vi "Setup Motors.vi"   [LabVIEW 2014]
uses:
  <vilib>/Rock Robotics/SystemInterfaces/Typedef/FPGA_TypedefDigitalModule.ctl
  <vilib>/Rock Robotics/SystemInterfaces/DIO/FPGA_DIOPWMChannel.ctl
  <vilib>/Rock Robotics/WPI/Joystick/WPI_JoystickDeviceEnum.ctl
  <vilib>/Rock Robotics/SystemInterfaces/Typedef/FPGA_TypedefAnalogModule.ctl
  <vilib>/Rock Robotics/SystemInterfaces/AI/FPGA_AIChannel.ctl
  <vilib>/Rock Robotics/WPI/Solenoid/WPI_SolenoidChannel.ctl
  <vilib>/Rock Robotics/SystemInterfaces/AI/FPGA_AIGyroChannel.ctl
  <vilib>/Rock Robotics/SystemInterfaces/Typedef/FPGA_TypedefAnalogModuleForGyro.ctl
  <vilib>/Rock Robotics/SystemInterfaces/DIO/FPGA_DIOChannel.ctl
  <vilib>/Rock Robotics/WPI/SafetyOutput/WPI_SafetyOutputConfigMenu.ctl
  <vilib>/Rock Robotics/WPI/MotorControl/WPI_MotorControlOpen Talon.vi
  <vilib>/Rock Robotics/WPI/Solenoid/WPI_SolenoidOpenSingle.vi
  <vilib>/Rock Robotics/WPI/Switch/WPI_SwitchOpenLimit.vi
  <vilib>/Rock Robotics/WPI/Counter/WPI_CounterDigitalInputToDigitalSource.vi
  Global Variables.vi
types:
  T1 = typedef "WPI_SafetyOutputConfigMenu.ctl" = enum16{"Enable", "Disable"}
  T2 = typedef "WPI_SolenoidChannel.ctl" = enum8{"Solenoid 0", "Solenoid 1", "Solenoid 2", "Solenoid 3", "Solenoid 4", "Solenoid 5", "Solenoid 6", "Solenoid 7", "Invalid"}
  T3 = typedef "FPGA_DIOChannel.ctl" = enum8{"DIO 0", "DIO 1", "DIO 2", "DIO 3", "DIO 4", "DIO 5", "DIO 6", "DIO 7", "DIO 8", "DIO 9", "DIO MXP 0", "DIO MXP 1", "DIO MXP 2", "DIO MXP 3", "DIO MXP 4", "DIO MXP 5", "DIO MXP 6", "DIO MXP 7", "DIO MXP 8", "DIO MXP 9", "DIO MXP 10", "DIO MXP 11", "DIO MXP 12", "DIO MXP 13", "DIO MXP 14", "DIO MXP 15", "Invalid"}
  T4 = typedef "FPGA_TypedefDigitalModule.ctl" = enum16{"Controller 1"}
  T5 = typedef "FPGA_TypedefAnalogModuleForGyro.ctl" = enum16{"Controller 1"}
  T6 = typedef "FPGA_AIGyroChannel.ctl" = enum8{"AI 0", "AI 1", "Invalid"}
  T7 = typedef "FPGA_DIOPWMChannel.ctl" = enum8{"PWM 0", "PWM 1", "PWM 2", "PWM 3", "PWM 4", "PWM 5", "PWM 6", "PWM 7", "PWM 8", "PWM 9", "PWM MXP 0", "PWM MXP 1", "PWM MXP 2", "PWM MXP 3", "PWM MXP 4", "PWM MXP 5", "PWM MXP 6", "PWM MXP 7", "PWM MXP 8", "PWM MXP 9", "Invalid"}
  T8 = typedef "FPGA_AIChannel.ctl" = enum8{"AI 0", "AI 1", "AI 2", "AI 3", "AI MXP 0", "AI MXP 1", "AI MXP 2", "AI MXP 3", "Invalid"}
  T9 = typedef "FPGA_TypedefAnalogModule.ctl" = enum16{"Controller 1"}
  T10 = typedef "WPI_JoystickDeviceEnum.ctl" = enum16{"USB 0", "USB 1", "USB 2", "USB 3", "USB 4", "USB 5"}
  T11 = typedef "WPI_MotorControlDeviceRef.ctl" = cluster{"DeviceStatus":errorcluster, "Type":T12, "PWM":cluster{"Controller":T4, "PWM Channel":T7, "DeadBand":T13}, "CAN":cluster{"Device Number":u8, "Control Mode":T14, "Semaphore":T15, "Max Vout":dbl, "TalonSRX Control Mode":T16}, "Invert":bool, "TransformRef":T17, "InvTransformRef":T17}
  T12 = typedef "WPI_MotorControlType.ctl" = enum16{"PWM", "CAN", "CANTalonSRX"}
  T13 = typedef "WPI_PWMDeadband.ctl" = cluster{"Name":string, "maxPositivePwm":i32, "minPositivePwm":i32, "centerPwm":i32, "maxNegativePwm":i32, "minNegativePwm":i32, "angularRange":u16}
  T14 = typedef "WPI_CANJaguar_ControlMode.ctl" = enum8{"Percent VBus", "Current", "Speed", "Position", "Voltage"}
  T15 = typedef "Semaphore RefNum" = refnum<k1>
  T16 = typedef "WPI_CANTalonSRX_APIControlMode.ctl" = enum8{"Percent VBus", "Speed", "Position", "Slave", "Unchanged / Invalid"}
  T17 = typedef "WPI_PWMTransform_ConPane.ctl" = refnum<vi>
  T18 = typedef "WPI_GyroDevRef.ctl" = cluster{"DevStatus":errorcluster, "Analog Module":T9, "Analog Channel":T8, "Offset":dbl, "Gain (VoltsPerDegree/Second)":dbl}
  T19 = typedef "WPI_SolenoidDevRef.ctl" = cluster{"DevStatus":errorcluster, "Pneumatics Control Module":u8, "Forward Solenoid Channel":T2, "Reverse Solenoid Channel":T2}
  T20 = typedef "WPI_SwitchDevRef.ctl" = cluster{"DevStatus":errorcluster, "DIO Channel":T3, "Controller":T4, "CntIndex":T21, "Normally Closed":bool}
  T21 = typedef "FPGA_CounterCtrSystemIndex.ctl" = enum8{"Ctr 0", "Ctr 1", "Ctr 2", "Ctr 3", "Ctr 4", "Ctr 5", "Ctr 6", "Ctr 7", "Invalid"}
  T22 = typedef "WPI_DigitalInputDevRef.ctl" = cluster{"DevStatus":errorcluster, "DIO Channel":T3, "Controller":T4}
  T23 = typedef "FPGA_CounterEncoderSourceConvertionLVSourceType.ctl" = cluster{"DevStatus":errorcluster, "AnalogTriggerMode?":bool, "DigitalMode":cluster{"Controller":T4, "DIO Channel":T24}, "AnalogTriggerMode":cluster{"AnalogTriggerIndex":T25, "OutputType":T26}}
  T24 = typedef "FPGA_DIODigitalSourceChannel.ctl" = enum8{"DIO 0", "DIO 1", "DIO 2", "DIO 3", "DIO 4", "DIO 5", "DIO 6", "DIO 7", "DIO 8", "DIO 9", "DIO MXP 0", "DIO MXP 1", "DIO MXP 2", "DIO MXP 3", "DIO MXP 4", "DIO MXP 5", "DIO MXP 6", "DIO MXP 7", "DIO MXP 8", "DIO MXP 9", "DIO MXP 10", "DIO MXP 11", "DIO MXP 12", "DIO MXP 13", "DIO MXP 14", "DIO MXP 15", "Disabled"}
  T25 = typedef "FPGA_AnalogTriggerIndex.ctl" = enum8{"Trig 0", "Trig 1", "Trig 2", "Trig 3", "Trig 4", "Trig 5", "Trig 6", "Trig 7", "Invalid"}
  T26 = typedef "FPGA_AnalogTriggerOutType.ctl" = enum16{"InWindow", "TriggerState", "Rising", "Falling"}
  T27 = typedef "WPI_AnalogChannelDevRef.ctl" = cluster{"DevStatus":errorcluster, "Controller":T9, "Analog Channel":T8}
  T28 = typedef "WPI_EncoderDevRef.ctl" = cluster{"DevStatus":errorcluster, "EncoderIndex":T29, "CounterIndex":T21, "DistancePerCount":dbl, "Decoding Type":T30}
  T29 = typedef "FPGA_EncoderIdx.ctl" = enum8{"Enc 0", "Enc 1", "Enc 2", "Enc 3", "Enc 4", "Enc 5", "Enc 6", "Enc 7", "Invalid"}
  T30 = typedef "WPI_EncoderType.ctl" = enum16{"1x", "2x", "4x"}
  T31 = typedef "WPI_JoystickDevRef.ctl" = cluster{"Device":T10}
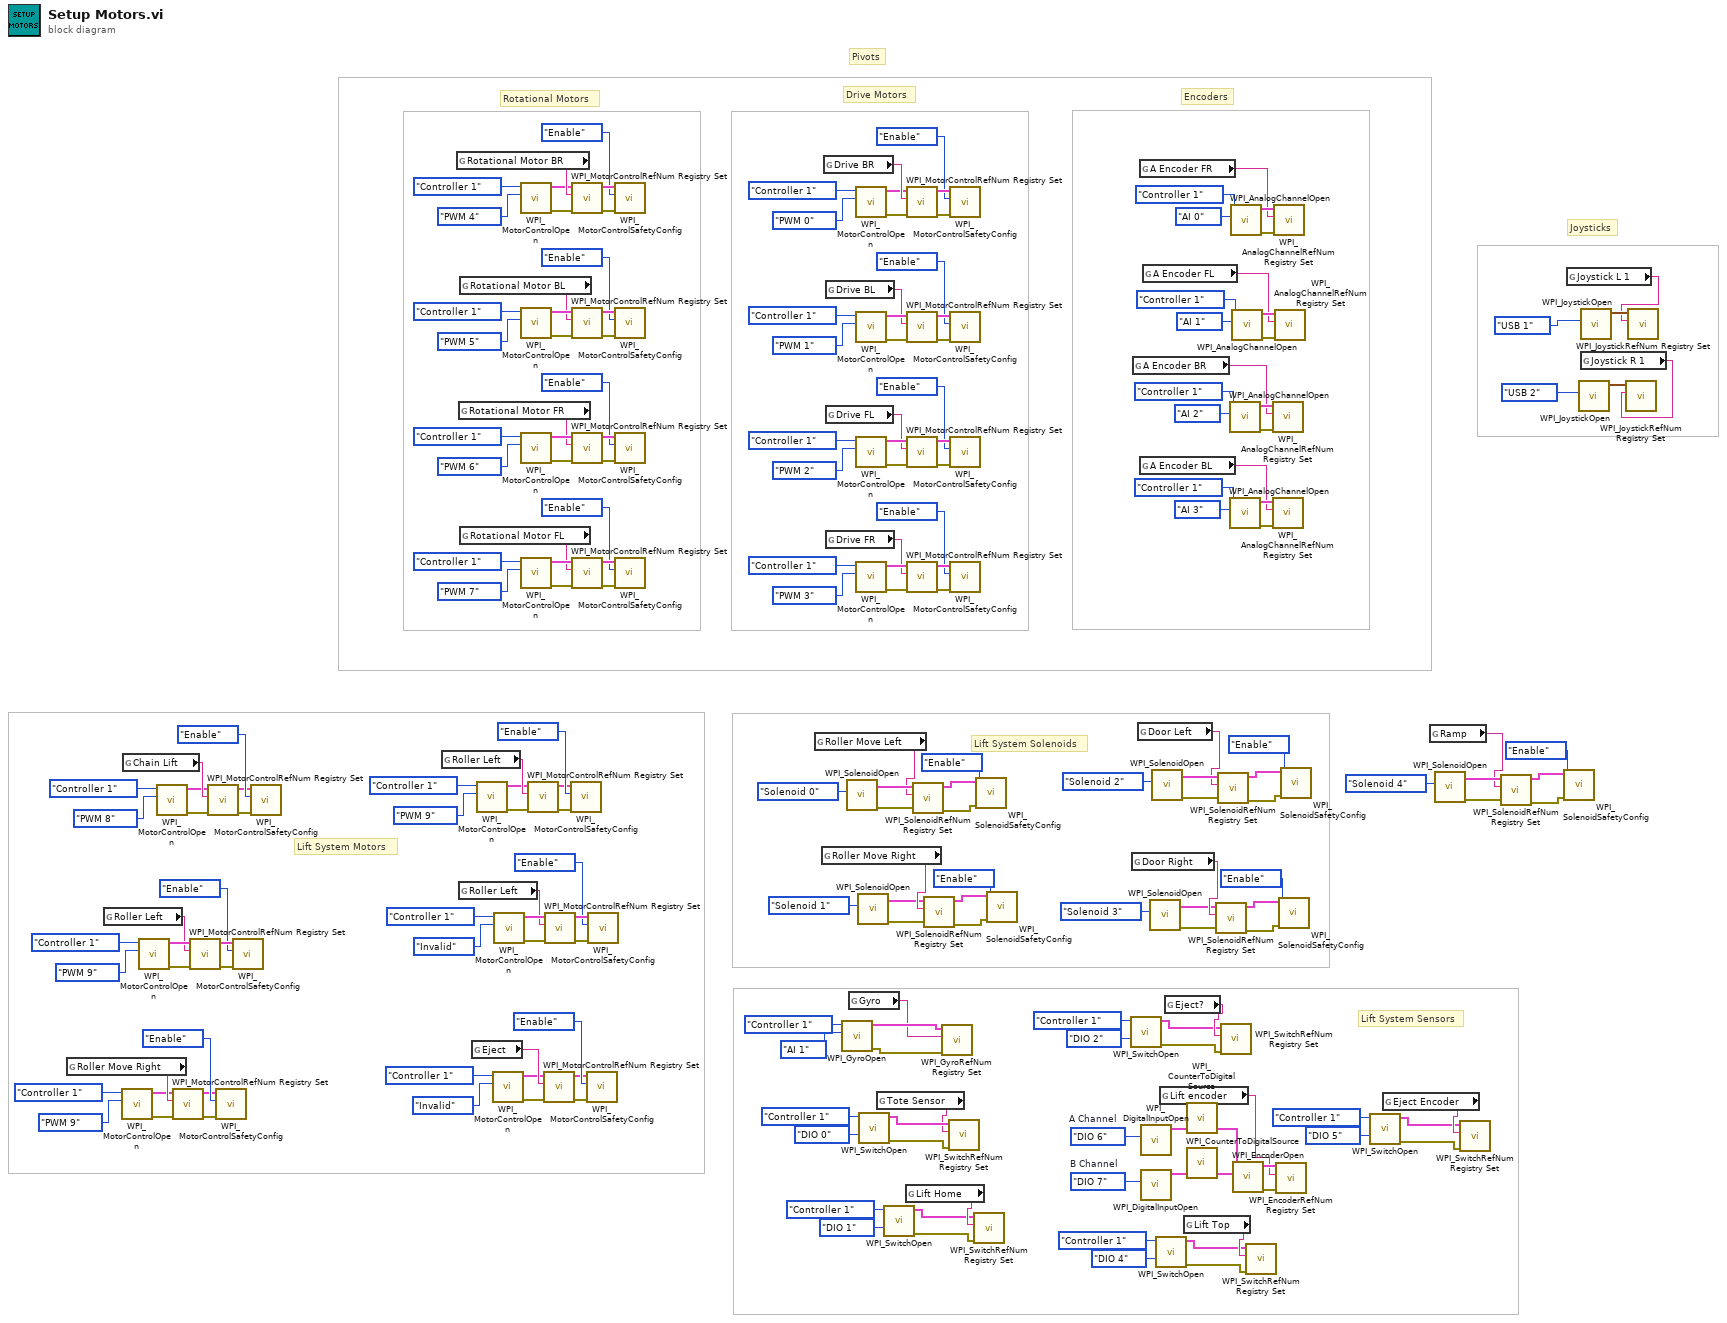
[diagram p0: block diagram]
diagram:
  w16 = FPGA_DIOChannel."DIO 7"  # B Channel
  w15 = FPGA_DIOChannel."DIO 6"  # A Channel
  # "Lift System Sensors"
  # "Lift System Solenoids"
  # "Lift System Motors"
  # "Encoders"
  # "Joysticks"
  # "Pivots"
  # "Rotational Motors"
  # "Drive Motors"
  n1 = global read "Global Variables.vi" "Roller Move Right"() -> (w105:string)
  n2 = global read "Global Variables.vi" "Roller Left"() -> (w108:string)
  n3 = call-poly <vilib>:"WPI_MotorControlOpen.vi"("PWM Channel"=FPGA_DIOPWMChannel."PWM 9", "Controller"=FPGA_TypedefDigitalModule."Controller 1") -> ("error out"=w100:errorcluster, "MotorControlDeviceRef"=w99:T11)  [unwired: 8 in]
  n4 = global read "Global Variables.vi" "Chain Lift"() -> (w121:string)
  n5 = call-poly <vilib>:"WPI_MotorControlOpen.vi"("PWM Channel"=FPGA_DIOPWMChannel."PWM 9", "Controller"=FPGA_TypedefDigitalModule."Controller 1") -> ("error out"=w113:errorcluster, "MotorControlDeviceRef"=w114:T11)  [unwired: 8 in]
  n6 = call-poly <vilib>:"WPI_MotorControlOpen.vi"("PWM Channel"=FPGA_DIOPWMChannel."PWM 8", "Controller"=FPGA_TypedefDigitalModule."Controller 1") -> ("error out"=w116:errorcluster, "MotorControlDeviceRef"=w115:T11)  [unwired: 8 in]
  n7 = call <vilib>:"WPI_MotorControlRefNum Registry Set.vi"("error in (no error)"=w100, "refnum name"=w105, "MotorControlDevRef"=w99) -> ("error out"=w102:errorcluster, "MotorControlDevRef"=w101:T11)  [unwired: 7 in]
  n8 = call <vilib>:"WPI_MotorControlRefNum Registry Set.vi"("error in (no error)"=w113, "refnum name"=w108, "MotorControlDevRef"=w114) -> ("error out"=w111:errorcluster, "MotorControlDevRef"=w112:T11)  [unwired: 7 in]
  n9 = call <vilib>:"WPI_MotorControlRefNum Registry Set.vi"("error in (no error)"=w116, "refnum name"=w121, "MotorControlDevRef"=w115) -> ("error out"=w118:errorcluster, "MotorControlDevRef"=w117:T11)  [unwired: 7 in]
  n10 = call <vilib>:"WPI_MotorControlSafetyConfig.vi"("error in (no error)"=w102, "mode"=WPI_SafetyOutputConfigMenu."Enable", "MotorControlDevRef"=w101) -> ()  [unwired: 7 in, 2 out]
  n11 = call <vilib>:"WPI_MotorControlSafetyConfig.vi"("error in (no error)"=w111, "mode"=WPI_SafetyOutputConfigMenu."Enable", "MotorControlDevRef"=w112) -> ()  [unwired: 7 in, 2 out]
  n12 = call <vilib>:"WPI_MotorControlSafetyConfig.vi"("error in (no error)"=w118, "mode"=WPI_SafetyOutputConfigMenu."Enable", "MotorControlDevRef"=w117) -> ()  [unwired: 7 in, 2 out]
  n13 = global read "Global Variables.vi" "Roller Left"() -> (w97:string)
  n14 = global read "Global Variables.vi" "Rotational Motor BR"() -> (w175:string)
  n15 = global read "Global Variables.vi" "Rotational Motor FR"() -> (w149:string)
  n16 = global read "Global Variables.vi" "Roller Left"() -> (w84:string)
  n17 = global read "Global Variables.vi" "Rotational Motor BL"() -> (w150:string)
  n18 = global read "Global Variables.vi" "Rotational Motor FL"() -> (w148:string)
  n19 = global read "Global Variables.vi" "Eject"() -> (w81:string)
  n20 = call-poly <vilib>:"WPI_MotorControlOpen.vi"("PWM Channel"=FPGA_DIOPWMChannel."PWM 9", "Controller"=FPGA_TypedefDigitalModule."Controller 1") -> ("error out"=w92:errorcluster, "MotorControlDeviceRef"=w91:T11)  [unwired: 8 in]
  n21 = call-poly <vilib>:"WPI_MotorControlOpen.vi"("PWM Channel"=FPGA_DIOPWMChannel."Invalid", "Controller"=FPGA_TypedefDigitalModule."Controller 1") -> ("error out"=w76:errorcluster, "MotorControlDeviceRef"=w75:T11)  [unwired: 8 in]
  n22 = call-poly <vilib>:"WPI_MotorControlOpen.vi"("PWM Channel"=FPGA_DIOPWMChannel."Invalid", "Controller"=FPGA_TypedefDigitalModule."Controller 1") -> ("error out"=w89:errorcluster, "MotorControlDeviceRef"=w90:T11)  [unwired: 8 in]
  n23 = call-poly <vilib>:"WPI_MotorControlOpen.vi"("PWM Channel"=FPGA_DIOPWMChannel."PWM 4", "Controller"=FPGA_TypedefDigitalModule."Controller 1") -> ("error out"=w173:errorcluster, "MotorControlDeviceRef"=w174:T11)  [unwired: 8 in]
  n24 = call-poly <vilib>:"WPI_MotorControlOpen.vi"("PWM Channel"=FPGA_DIOPWMChannel."PWM 5", "Controller"=FPGA_TypedefDigitalModule."Controller 1") -> ("error out"=w167:errorcluster, "MotorControlDeviceRef"=w168:T11)  [unwired: 8 in]
  n25 = call-poly <vilib>:"WPI_MotorControlOpen.vi"("PWM Channel"=FPGA_DIOPWMChannel."PWM 6", "Controller"=FPGA_TypedefDigitalModule."Controller 1") -> ("error out"=w161:errorcluster, "MotorControlDeviceRef"=w162:T11)  [unwired: 8 in]
  n26 = call-poly <vilib>:"WPI_MotorControlOpen.vi"("PWM Channel"=FPGA_DIOPWMChannel."PWM 7", "Controller"=FPGA_TypedefDigitalModule."Controller 1") -> ("error out"=w155:errorcluster, "MotorControlDeviceRef"=w156:T11)  [unwired: 8 in]
  n27 = call <vilib>:"WPI_MotorControlRefNum Registry Set.vi"("error in (no error)"=w92, "refnum name"=w97, "MotorControlDevRef"=w91) -> ("error out"=w94:errorcluster, "MotorControlDevRef"=w93:T11)  [unwired: 7 in]
  n28 = call <vilib>:"WPI_MotorControlRefNum Registry Set.vi"("error in (no error)"=w76, "refnum name"=w81, "MotorControlDevRef"=w75) -> ("error out"=w78:errorcluster, "MotorControlDevRef"=w77:T11)  [unwired: 7 in]
  n29 = call <vilib>:"WPI_MotorControlRefNum Registry Set.vi"("error in (no error)"=w89, "refnum name"=w84, "MotorControlDevRef"=w90) -> ("error out"=w87:errorcluster, "MotorControlDevRef"=w88:T11)  [unwired: 7 in]
  n30 = call <vilib>:"WPI_MotorControlSafetyConfig.vi"("error in (no error)"=w94, "mode"=WPI_SafetyOutputConfigMenu."Enable", "MotorControlDevRef"=w93) -> ()  [unwired: 7 in, 2 out]
  n31 = call <vilib>:"WPI_MotorControlRefNum Registry Set.vi"("error in (no error)"=w173, "refnum name"=w175, "MotorControlDevRef"=w174) -> ("error out"=w171:errorcluster, "MotorControlDevRef"=w172:T11)  [unwired: 7 in]
  n32 = call <vilib>:"WPI_MotorControlRefNum Registry Set.vi"("error in (no error)"=w167, "refnum name"=w150, "MotorControlDevRef"=w168) -> ("error out"=w165:errorcluster, "MotorControlDevRef"=w166:T11)  [unwired: 7 in]
  n33 = call <vilib>:"WPI_MotorControlRefNum Registry Set.vi"("error in (no error)"=w161, "refnum name"=w149, "MotorControlDevRef"=w162) -> ("error out"=w159:errorcluster, "MotorControlDevRef"=w160:T11)  [unwired: 7 in]
  n34 = call <vilib>:"WPI_MotorControlRefNum Registry Set.vi"("error in (no error)"=w155, "refnum name"=w148, "MotorControlDevRef"=w156) -> ("error out"=w153:errorcluster, "MotorControlDevRef"=w154:T11)  [unwired: 7 in]
  n35 = call <vilib>:"WPI_MotorControlSafetyConfig.vi"("error in (no error)"=w78, "mode"=WPI_SafetyOutputConfigMenu."Enable", "MotorControlDevRef"=w77) -> ()  [unwired: 7 in, 2 out]
  n36 = call <vilib>:"WPI_MotorControlSafetyConfig.vi"("error in (no error)"=w87, "mode"=WPI_SafetyOutputConfigMenu."Enable", "MotorControlDevRef"=w88) -> ()  [unwired: 7 in, 2 out]
  n37 = call <vilib>:"WPI_MotorControlSafetyConfig.vi"("error in (no error)"=w171, "mode"=WPI_SafetyOutputConfigMenu."Enable", "MotorControlDevRef"=w172) -> ()  [unwired: 7 in, 2 out]
  n38 = call <vilib>:"WPI_MotorControlSafetyConfig.vi"("error in (no error)"=w165, "mode"=WPI_SafetyOutputConfigMenu."Enable", "MotorControlDevRef"=w166) -> ()  [unwired: 7 in, 2 out]
  n39 = call <vilib>:"WPI_MotorControlSafetyConfig.vi"("error in (no error)"=w159, "mode"=WPI_SafetyOutputConfigMenu."Enable", "MotorControlDevRef"=w160) -> ()  [unwired: 7 in, 2 out]
  n40 = call <vilib>:"WPI_MotorControlSafetyConfig.vi"("error in (no error)"=w153, "mode"=WPI_SafetyOutputConfigMenu."Enable", "MotorControlDevRef"=w154) -> ()  [unwired: 7 in, 2 out]
  n41 = global read "Global Variables.vi" "Roller Move Left"() -> (w69:string)
  n42 = global read "Global Variables.vi" "Roller Move Right"() -> (w68:string)
  n43 = global read "Global Variables.vi" "Drive BR"() -> (w212:string)
  n44 = global read "Global Variables.vi" "Drive BL"() -> (w187:string)
  n45 = global read "Global Variables.vi" "Drive FL"() -> (w186:string)
  n46 = global read "Global Variables.vi" "Drive FR"() -> (w185:string)
  n47 = call <vilib>:"WPI_GyroOpen.vi"("Analog Channel"=FPGA_AIGyroChannel."AI 1", "Controller"=FPGA_TypedefAnalogModuleForGyro."Controller 1") -> ("error out"=w49:errorcluster, "GyroDevRef"=w50:T18)  [unwired: 7 in, 1 out]
  n48 = call-poly <vilib>:"WPI_SolenoidOpen.vi"("Solenoid Channel"=WPI_SolenoidChannel."Solenoid 0") -> ("error out"=w71:errorcluster, "SolenoidDevRef"=w72:T19)  [unwired: 9 in]
  n49 = global read "Global Variables.vi" "Gyro"() -> (w46:string)
  n50 = call-poly <vilib>:"WPI_MotorControlOpen.vi"("PWM Channel"=FPGA_DIOPWMChannel."PWM 0", "Controller"=FPGA_TypedefDigitalModule."Controller 1") -> ("error out"=w210:errorcluster, "MotorControlDeviceRef"=w211:T11)  [unwired: 8 in]
  n51 = call-poly <vilib>:"WPI_MotorControlOpen.vi"("PWM Channel"=FPGA_DIOPWMChannel."PWM 1", "Controller"=FPGA_TypedefDigitalModule."Controller 1") -> ("error out"=w204:errorcluster, "MotorControlDeviceRef"=w205:T11)  [unwired: 8 in]
  n52 = call-poly <vilib>:"WPI_MotorControlOpen.vi"("PWM Channel"=FPGA_DIOPWMChannel."PWM 2", "Controller"=FPGA_TypedefDigitalModule."Controller 1") -> ("error out"=w198:errorcluster, "MotorControlDeviceRef"=w199:T11)  [unwired: 8 in]
  n53 = call-poly <vilib>:"WPI_MotorControlOpen.vi"("PWM Channel"=FPGA_DIOPWMChannel."PWM 3", "Controller"=FPGA_TypedefDigitalModule."Controller 1") -> ("error out"=w192:errorcluster, "MotorControlDeviceRef"=w193:T11)  [unwired: 8 in]
  n54 = call-poly <vilib>:"WPI_SolenoidOpen.vi"("Solenoid Channel"=WPI_SolenoidChannel."Solenoid 1") -> ("error out"=w66:errorcluster, "SolenoidDevRef"=w65:T19)  [unwired: 9 in]
  n55 = call-poly <vilib>:"WPI_SwitchOpen.vi"("DIO Channel"=FPGA_DIOChannel."DIO 0", "Controller"=FPGA_TypedefDigitalModule."Controller 1") -> ("error out"=w44:errorcluster, "SwitchDevRef"=w45:T20)  [unwired: 8 in]
  n56 = global read "Global Variables.vi" "Tote Sensor"() -> (w41:string)
  n57 = call-poly <vilib>:"WPI_SwitchOpen.vi"("DIO Channel"=FPGA_DIOChannel."DIO 1", "Controller"=FPGA_TypedefDigitalModule."Controller 1") -> ("error out"=w37:errorcluster, "SwitchDevRef"=w36:T20)  [unwired: 8 in]
  n58 = global read "Global Variables.vi" "Lift Home"() -> (w40:string)
  n59 = call <vilib>:"WPI_MotorControlRefNum Registry Set.vi"("error in (no error)"=w210, "refnum name"=w212, "MotorControlDevRef"=w211) -> ("error out"=w208:errorcluster, "MotorControlDevRef"=w209:T11)  [unwired: 7 in]
  n60 = call <vilib>:"WPI_MotorControlRefNum Registry Set.vi"("error in (no error)"=w204, "refnum name"=w187, "MotorControlDevRef"=w205) -> ("error out"=w202:errorcluster, "MotorControlDevRef"=w203:T11)  [unwired: 7 in]
  n61 = call <vilib>:"WPI_MotorControlRefNum Registry Set.vi"("error in (no error)"=w198, "refnum name"=w186, "MotorControlDevRef"=w199) -> ("error out"=w196:errorcluster, "MotorControlDevRef"=w197:T11)  [unwired: 7 in]
  n62 = call <vilib>:"WPI_MotorControlRefNum Registry Set.vi"("error in (no error)"=w192, "refnum name"=w185, "MotorControlDevRef"=w193) -> ("error out"=w190:errorcluster, "MotorControlDevRef"=w191:T11)  [unwired: 7 in]
  n63 = call <vilib>:"WPI_SolenoidRefNum Registry Set.vi"("error in (no error)"=w71, "refnum name"=w69, "SolenoidDevRef"=w72) -> ("error out"=w73:errorcluster, "SolenoidDevRef"=w74:T19)  [unwired: 7 in]
  n64 = call <vilib>:"WPI_SolenoidRefNum Registry Set.vi"("error in (no error)"=w66, "refnum name"=w68, "SolenoidDevRef"=w65) -> ("error out"=w64:errorcluster, "SolenoidDevRef"=w63:T19)  [unwired: 7 in]
  n65 = call <vilib>:"WPI_GyroRefNum Registry Set.vi"("error in (no error)"=w49, "refnum name"=w46, "GyroDevRef"=w50) -> ()  [unwired: 7 in, 2 out]
  n66 = call <vilib>:"WPI_SwitchRefNum Registry Set.vi"("error in (no error)"=w44, "refnum name"=w41, "SwitchDevRef"=w45) -> ()  [unwired: 7 in, 2 out]
  n67 = call <vilib>:"WPI_MotorControlSafetyConfig.vi"("error in (no error)"=w208, "mode"=WPI_SafetyOutputConfigMenu."Enable", "MotorControlDevRef"=w209) -> ()  [unwired: 7 in, 2 out]
  n68 = call <vilib>:"WPI_MotorControlSafetyConfig.vi"("error in (no error)"=w202, "mode"=WPI_SafetyOutputConfigMenu."Enable", "MotorControlDevRef"=w203) -> ()  [unwired: 7 in, 2 out]
  n69 = call <vilib>:"WPI_MotorControlSafetyConfig.vi"("error in (no error)"=w196, "mode"=WPI_SafetyOutputConfigMenu."Enable", "MotorControlDevRef"=w197) -> ()  [unwired: 7 in, 2 out]
  n70 = call <vilib>:"WPI_MotorControlSafetyConfig.vi"("error in (no error)"=w190, "mode"=WPI_SafetyOutputConfigMenu."Enable", "MotorControlDevRef"=w191) -> ()  [unwired: 7 in, 2 out]
  n71 = call <vilib>:"WPI_SwitchRefNum Registry Set.vi"("error in (no error)"=w37, "refnum name"=w40, "SwitchDevRef"=w36) -> ()  [unwired: 7 in, 2 out]
  n72 = call <vilib>:"WPI_SolenoidSafetyConfig.vi"("error in (no error)"=w73, "mode"=WPI_SafetyOutputConfigMenu."Enable", "SolenoidDevRef"=w74) -> ()  [unwired: 7 in, 2 out]
  n73 = call <vilib>:"WPI_SolenoidSafetyConfig.vi"("error in (no error)"=w64, "mode"=WPI_SafetyOutputConfigMenu."Enable", "SolenoidDevRef"=w63) -> ()  [unwired: 7 in, 2 out]
  n74 = call-poly <vilib>:"WPI_SwitchOpen.vi"("DIO Channel"=FPGA_DIOChannel."DIO 2", "Controller"=FPGA_TypedefDigitalModule."Controller 1") -> ("error out"=w27:errorcluster, "SwitchDevRef"=w26:T20)  [unwired: 8 in]
  n75 = global read "Global Variables.vi" "Door Right"() -> (w56:string)
  n76 = global read "Global Variables.vi" "A Encoder BR"() -> (w124:string)
  n77 = global read "Global Variables.vi" "Door Left"() -> (w57:string)
  n78 = global read "Global Variables.vi" "A Encoder FR"() -> (w126:string)
  n79 = global read "Global Variables.vi" "A Encoder BL"() -> (w125:string)
  n80 = call <vilib>:"WPI_DigitalInputOpen.vi"("DIO Channel"=w15) -> ("DigitalInputDevRef"=w12:T22)  [unwired: 2 in, 8 out]
  n81 = call <vilib>:"WPI_DigitalInputOpen.vi"("DIO Channel"=w16) -> ("DigitalInputDevRef"=w13:T22)  [unwired: 2 in, 8 out]
  n82 = global read "Global Variables.vi" "A Encoder FL"() -> (w123:string)
  n83 = call-poly <vilib>:"WPI_SolenoidOpen.vi"("Solenoid Channel"=WPI_SolenoidChannel."Solenoid 3") -> ("error out"=w54:errorcluster, "SolenoidDevRef"=w53:T19)  [unwired: 9 in]
  n84 = call-poly <vilib>:"WPI_SolenoidOpen.vi"("Solenoid Channel"=WPI_SolenoidChannel."Solenoid 2") -> ("error out"=w59:errorcluster, "SolenoidDevRef"=w60:T19)  [unwired: 9 in]
  n85 = call-poly <vilib>:"WPI_SwitchOpen.vi"("DIO Channel"=FPGA_DIOChannel."DIO 4", "Controller"=FPGA_TypedefDigitalModule."Controller 1") -> ("error out"=w32:errorcluster, "SwitchDevRef"=w31:T20)  [unwired: 8 in]
  n86 = global read "Global Variables.vi" "Lift encoder"() -> (w8:string)
  n87 = global read "Global Variables.vi" "Eject?"() -> (w30:string)
  n88 = global read "Global Variables.vi" "Lift Top"() -> (w35:string)
  n89 = call-poly <vilib>:"WPI_CounterToDigitalSource.vi"("DigitalInputDevRef"=w12) -> ("Digital Source"=w11:T23)  [unwired: 6 out]
  n90 = call-poly <vilib>:"WPI_CounterToDigitalSource.vi"("DigitalInputDevRef"=w13) -> ("Digital Source"=w14:T23)  [unwired: 6 out]
  n91 = call <vilib>:"WPI_SolenoidRefNum Registry Set.vi"("error in (no error)"=w54, "refnum name"=w56, "SolenoidDevRef"=w53) -> ("error out"=w52:errorcluster, "SolenoidDevRef"=w51:T19)  [unwired: 7 in]
  n92 = call <vilib>:"WPI_SolenoidRefNum Registry Set.vi"("error in (no error)"=w59, "refnum name"=w57, "SolenoidDevRef"=w60) -> ("error out"=w61:errorcluster, "SolenoidDevRef"=w62:T19)  [unwired: 7 in]
  n93 = call <vilib>:"WPI_SwitchRefNum Registry Set.vi"("error in (no error)"=w27, "refnum name"=w30, "SwitchDevRef"=w26) -> ()  [unwired: 7 in, 2 out]
  n94 = call <vilib>:"WPI_AnalogChannelOpen.vi"("Analog Channel"=FPGA_AIChannel."AI 2", "Controller"=FPGA_TypedefAnalogModule."Controller 1") -> ("error out"=w133:errorcluster, "AIDeviceRef"=w134:T27)  [unwired: 8 in]
  n95 = call <vilib>:"WPI_AnalogChannelOpen.vi"("Analog Channel"=FPGA_AIChannel."AI 3", "Controller"=FPGA_TypedefAnalogModule."Controller 1") -> ("error out"=w129:errorcluster, "AIDeviceRef"=w130:T27)  [unwired: 8 in]
  n96 = call <vilib>:"WPI_AnalogChannelOpen.vi"("Analog Channel"=FPGA_AIChannel."AI 0", "Controller"=FPGA_TypedefAnalogModule."Controller 1") -> ("error out"=w141:errorcluster, "AIDeviceRef"=w142:T27)  [unwired: 8 in]
  n97 = call <vilib>:"WPI_AnalogChannelOpen.vi"("Analog Channel"=FPGA_AIChannel."AI 1", "Controller"=FPGA_TypedefAnalogModule."Controller 1") -> ("error out"=w137:errorcluster, "AIDeviceRef"=w138:T27)  [unwired: 8 in]
  n98 = call <vilib>:"WPI_EncoderOpen.vi"("BSource"=w14, "ASource"=w11) -> ("error out"=w10:errorcluster, "EncoderDevRef"=w9:T28)  [unwired: 6 in, 2 out]
  n99 = call <vilib>:"WPI_SwitchRefNum Registry Set.vi"("error in (no error)"=w32, "refnum name"=w35, "SwitchDevRef"=w31) -> ()  [unwired: 7 in, 2 out]
  n100 = call <vilib>:"WPI_AnalogChannelRefNum Registry Set.vi"("error in (no error)"=w133, "refnum name"=w124, "AIDeviceRef"=w134) -> ()  [unwired: 7 in, 2 out]
  n101 = call <vilib>:"WPI_AnalogChannelRefNum Registry Set.vi"("error in (no error)"=w129, "refnum name"=w125, "AIDeviceRef"=w130) -> ()  [unwired: 7 in, 2 out]
  n102 = call <vilib>:"WPI_AnalogChannelRefNum Registry Set.vi"("error in (no error)"=w141, "refnum name"=w126, "AIDeviceRef"=w142) -> ()  [unwired: 7 in, 2 out]
  n103 = call <vilib>:"WPI_AnalogChannelRefNum Registry Set.vi"("error in (no error)"=w137, "refnum name"=w123, "AIDeviceRef"=w138) -> ()  [unwired: 7 in, 2 out]
  n104 = call <vilib>:"WPI_EncoderRefNum Registry Set.vi"("error in (no error)"=w10, "refnum name"=w8, "EncoderDevRef"=w9) -> ()  [unwired: 7 in, 2 out]
  n105 = call <vilib>:"WPI_SolenoidSafetyConfig.vi"("error in (no error)"=w52, "mode"=WPI_SafetyOutputConfigMenu."Enable", "SolenoidDevRef"=w51) -> ()  [unwired: 7 in, 2 out]
  n106 = call <vilib>:"WPI_SolenoidSafetyConfig.vi"("error in (no error)"=w61, "mode"=WPI_SafetyOutputConfigMenu."Enable", "SolenoidDevRef"=w62) -> ()  [unwired: 7 in, 2 out]
  n107 = call-poly <vilib>:"WPI_SwitchOpen.vi"("DIO Channel"=FPGA_DIOChannel."DIO 5", "Controller"=FPGA_TypedefDigitalModule."Controller 1") -> ("error out"=w22:errorcluster, "SwitchDevRef"=w21:T20)  [unwired: 8 in]
  n108 = global read "Global Variables.vi" "Eject Encoder"() -> (w25:string)
  n109 = global read "Global Variables.vi" "Ramp"() -> (w1:string)
  n110 = call-poly <vilib>:"WPI_SolenoidOpen.vi"("Solenoid Channel"=WPI_SolenoidChannel."Solenoid 4") -> ("error out"=w3:errorcluster, "SolenoidDevRef"=w4:T19)  [unwired: 9 in]
  n111 = call <vilib>:"WPI_SwitchRefNum Registry Set.vi"("error in (no error)"=w22, "refnum name"=w25, "SwitchDevRef"=w21) -> ()  [unwired: 7 in, 2 out]
  n112 = call <vilib>:"WPI_SolenoidRefNum Registry Set.vi"("error in (no error)"=w3, "refnum name"=w1, "SolenoidDevRef"=w4) -> ("error out"=w5:errorcluster, "SolenoidDevRef"=w6:T19)  [unwired: 7 in]
  n113 = call <vilib>:"WPI_SolenoidSafetyConfig.vi"("error in (no error)"=w5, "mode"=WPI_SafetyOutputConfigMenu."Enable", "SolenoidDevRef"=w6) -> ()  [unwired: 7 in, 2 out]
  n114 = global read "Global Variables.vi" "Joystick L 1"() -> (w179:string)
  n115 = call <vilib>:"WPI_JoystickOpen.vi"("JoystickDevice"=WPI_JoystickDeviceEnum."USB 2") -> ("JoystickDevRef"=w177:T31)  [unwired: 10 in]
  n116 = call <vilib>:"WPI_JoystickOpen.vi"("JoystickDevice"=WPI_JoystickDeviceEnum."USB 1") -> ("JoystickDevRef"=w180:T31)  [unwired: 10 in]
  n117 = global read "Global Variables.vi" "Joystick R 1"() -> (w176:string)
  n118 = call <vilib>:"WPI_JoystickRefNum Registry Set.vi"("refnum name"=w176, "JoystickDevRef"=w177) -> ()  [unwired: 8 in, 2 out]
  n119 = call <vilib>:"WPI_JoystickRefNum Registry Set.vi"("refnum name"=w179, "JoystickDevRef"=w180) -> ()  [unwired: 8 in, 2 out]
